vi "DriveEncoderConverter.vi"(2 "Mode":enum16{"Count -> Inches", "Inches -> Count"}(ring), 3 "Input":dbl) -> (1 "Output":dbl)   [LabVIEW 2018]
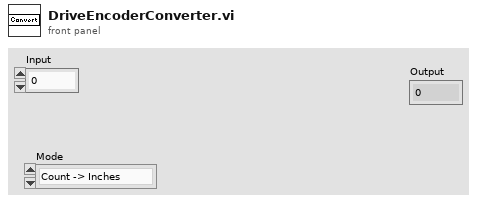
[diagram p1: front panel]
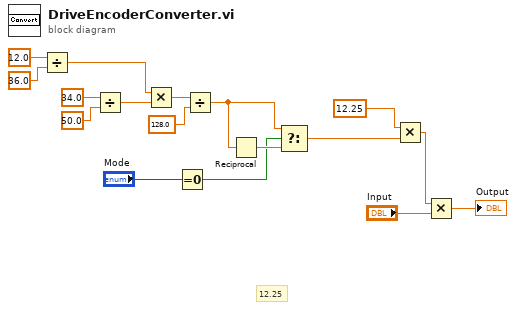
[diagram p0: block diagram]
diagram:
  # "12.25"
  n1 = Divide(x=12.0, y=36.0 ("x")) -> (x/y=w12:dbl)
  n2 = Divide(x=34.0, y=50.0 ("x")) -> (x/y=w13:dbl)
  n3 = Multiply(x=w12, y=w13) -> (x*y=w4:dbl)
  n4 = Equal To 0?(x="Mode") -> (x = 0?=w7:bool)
  n5 = Divide(x=w4, y=128.0 ("x")) -> (x/y=w2:dbl)
  n6 = Reciprocal(x=w2) -> (1/x=w11:dbl)
  n7 = Select(t=w2, s=w7, f=w11) -> (s? t:f=w6:dbl)
  n8 = Multiply(x=12.25, y=w6) -> (x*y=w5:dbl)
  n9 = Multiply(x=w5, y="Input") -> (x*y=→"Output":dbl)
